vi "ConnectLogin.vi"(8 "error in (no error)":errorcluster, 11 "Telnet in":refnum<class "Telnet.lvclass">) -> (0 "error out":errorcluster, 1 "Array":string[](array[string]), 2 "output":string, 3 "Telnet out":refnum<class "Telnet.lvclass">)   [LabVIEW 2011, in "Hardware.lvlib" / "HWControllers.lvlib" / "Telnet.lvclass"]
uses:
  Telnet.lvclass
  Telnet.lvclass/Telnet.ctl
  <vilib>/addons/internet/NI_InternetTK_Core_VIs.lvlib
panel:
  in  "stop":bool
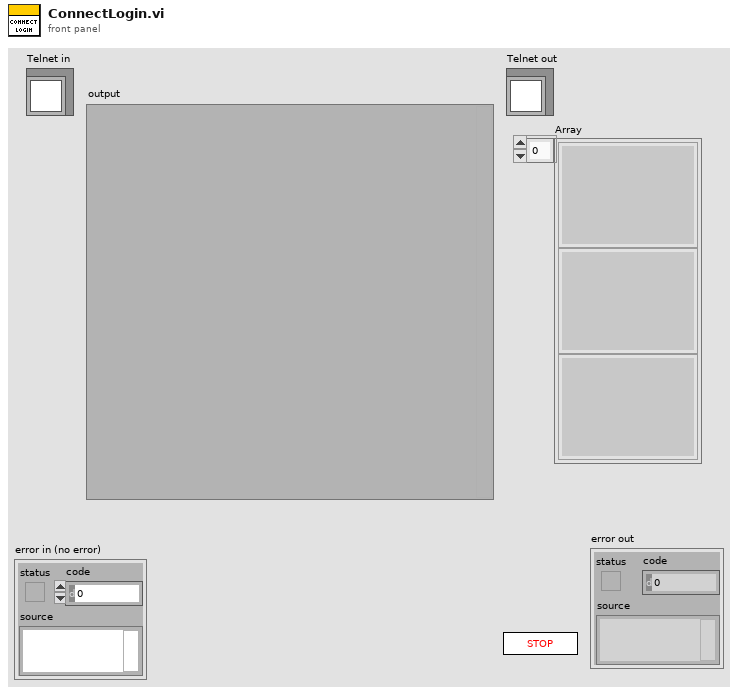
[diagram p1: front panel]
types:
  T1 = typedef "Telnet Session.ctl" = refnum<k1>
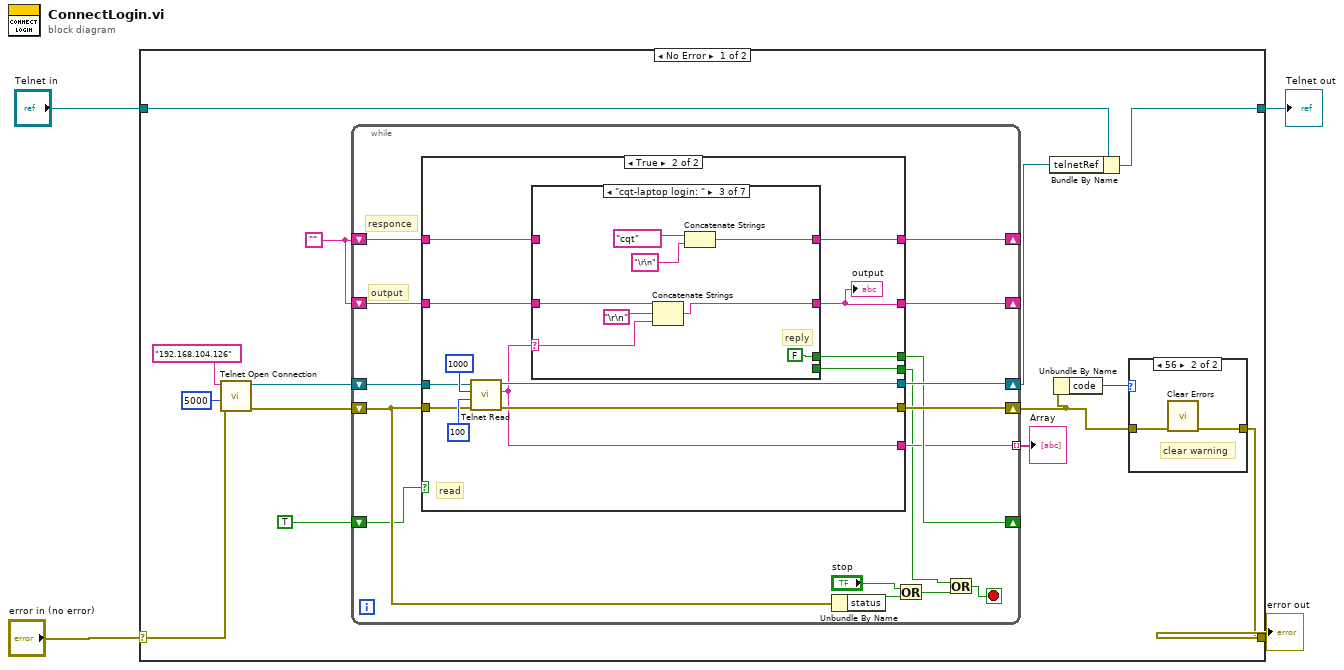
[diagram p0: block diagram]
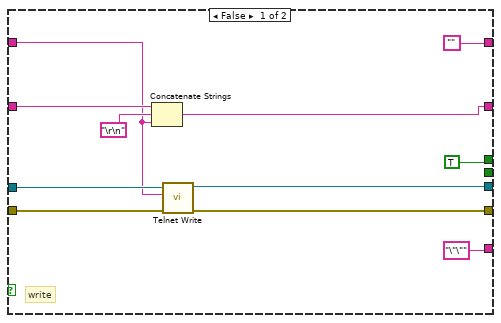
[diagram p3: hidden frame]
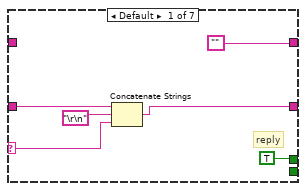
[diagram p4: hidden frame]
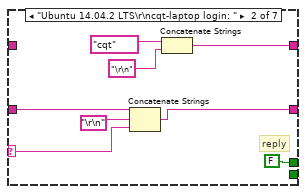
[diagram p5: hidden frame]
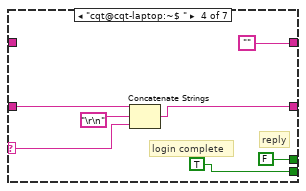
[diagram p6: hidden frame]
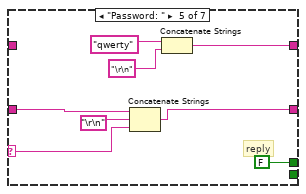
[diagram p7: hidden frame]
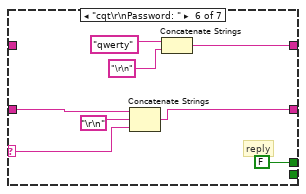
[diagram p8: hidden frame]
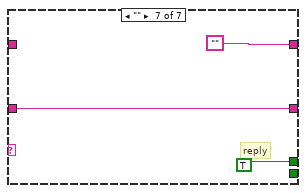
[diagram p9: hidden frame]
diagram:
  n1 = case shown="No Error" "error in (no error)" {
    selector: "error in (no error)" -> [w11 w111]
    tunnel: [w5 w111] -> w3
    tunnel: [w8 w110] -> w1
    tunnel: "Telnet in" -> [w9 w110]
    frame No Error {
      w15 = ""
      n2 = call <vilib>:"Telnet Open Connection.vi"("error in (no error)"=w11, "timeout ms (60000)"=5000, "address"="192.168.104.126" ("Address")) -> ("error out"=w13:errorcluster, "telnet connection"=w14:T1)  [unwired: 7 in]
      n3 = while {
        shift-right: [w36] -> w10
        shift-left: w14 -> [w37]
        shift-right: [w35] -> w6
        shift-left: w13 -> [w32]
        shift-right: [w30] -> _
        shift-left: w15 -> [w31]
        shift-right: [w28] -> _
        shift-left: TRUE -> [w29]
        shift-right: [w27] -> _
        shift-left: w15 -> [w26]
        tunnel: [w25] -> w12 mode=indexing
        stop <- w22 stop-if-true
        # "output"
        # "responce"
        n4 = case shown="True" w29 {
          tunnel: w37 -> [w47 w59]
          tunnel: [w44 w58] -> w36
          tunnel: [w45 w57] -> w35
          tunnel: w32 -> [w46 w56]
          tunnel: w31 -> [w42 w55]
          tunnel: [w41 w54] -> w30
          tunnel: [TRUE w53] -> w28
          tunnel: ["" w52] -> w27
          tunnel: w26 -> [w40 w51]
          tunnel: ["\"\"" w50] -> w25
          tunnel: [_ w49] -> w23
          frame False {
            # "write"
            n5 = Concatenate Strings(w42, "\r\n", w40) -> (w41:string)
            n6 = call <vilib>:"Telnet Write.vi"("error in (no error)"=w46, "data in"=w40, "telnet connection"=w47) -> ("error out"=w45:errorcluster, "telnet connection out"=w44:T1)  [unwired: 4 in, 1 out]
          }
          frame True {
            # "read"
            n7 = call <vilib>:"Telnet Read.vi"("error in (no error)"=w56, "timeout ms (25000)"=100, "bytes to read"=1000, "telnet connection"=w59) -> ("error out"=w57:errorcluster, "data out"=w50:string, "telnet connection out"=w58:T1)  [unwired: 3 out]
            n8 = case shown="\"cqt-laptop login: \"" w50 {
              selector: w50 -> [w64 w71 w79 w86 w94 w102 _]
              tunnel: w55 -> [w66 w73 w81 w88 w96 w104 w109]
              tunnel: [w65 w72 w80 w87 w95 w103 w109] -> w54
              tunnel: [TRUE FALSE FALSE FALSE FALSE FALSE TRUE] -> w53
              tunnel: ["" w68 w76 "" w91 w99 ""] -> w52
              tunnel: w51 -> [_ _ _ _ _ _ _]
              tunnel: [_ _ _ TRUE _ _ _] -> w49
              frame Default {
                # "reply"
                n9 = Concatenate Strings(w66, "\r\n", w64) -> (w65:string)
              }
              frame "Ubuntu 14.04.2 LTS\r\ncqt-laptop login: " {
                # "reply"
                n10 = Concatenate Strings(w73, "\r\n", w71) -> (w72:string)
                n11 = Concatenate Strings("cqt", "\r\n") -> (w68:string)
              }
              frame "cqt-laptop login: " {
                # "reply"
                n12 = Concatenate Strings(w81, "\r\n", w79) -> (w80:string)
                n13 = Concatenate Strings("cqt", "\r\n") -> (w76:string)
              }
              frame "cqt@cqt-laptop:~$ " {
                # "login complete"
                # "reply"
                n14 = Concatenate Strings(w88, "\r\n", w86) -> (w87:string)
              }
              frame "Password: " {
                # "reply"
                n15 = Concatenate Strings(w96, "\r\n", w94) -> (w95:string)
                n16 = Concatenate Strings("qwerty", "\r\n") -> (w91:string)
              }
              frame "cqt\r\nPassword: " {
                # "reply"
                n17 = Concatenate Strings(w104, "\r\n", w102) -> (w103:string)
                n18 = Concatenate Strings("qwerty", "\r\n") -> (w99:string)
              }
              frame "" {
                # "reply"
              }
            }
            "output" <- w54
          }
        }
        n19 = Unbundle By Name(w32) -> ("status"=w33:bool)
        n20 = Or(x="stop", y=w33) -> (x .or. y?=w24:bool)
        n21 = Or(x=w23, y=w24) -> (x .or. y?=w22:bool)
      }
      "Array" <- w12
      n22 = Bundle By Name(cluster=w9, "telnetRef"=w10) -> (w8:refnum<class "Telnet.lvclass">)
      n23 = Unbundle By Name(w6) -> ("code"=w7:i32)
      n24 = case shown="56" w7 {
        tunnel: w6 -> [w19 w21]
        tunnel: [w19 w20] -> w5
        frame 0, Default {
        }
        frame 56 {
          # "clear warning"
          n25 = call <vilib>:"Clear Errors.vi"("error in (no error)"=w21) -> ("error out"=w20:errorcluster)  [unwired: 6 in]
        }
      }
    }
    frame Error {
    }
  }
  "error out" <- w3
  "Telnet out" <- w1
